vi "ALTS-2015 OPC Engine Main.vi"(8 "error in (no error)":errorcluster) -> (0 "error out":errorcluster)   [LabVIEW 2013]
doc: "Copyright © 2005, Soliton Technologies.\nAll rights reserved."
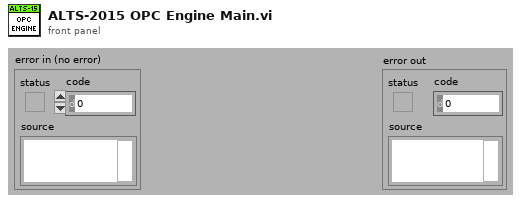
[diagram p1: front panel]
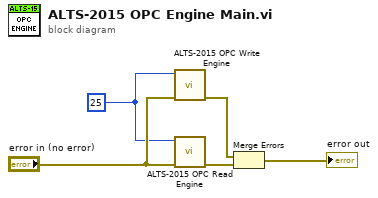
[diagram p0: block diagram]
diagram:
  w1 = u32 25 ("Delay (ms)")
  n1 = call "ALTS-2015 OPC Write Engine.vi"("error in (no error)"="error in (no error)", "Delay (ms)"=w1) -> ("error out"=w4:errorcluster)  [unwired: 9 in]
  n2 = call "ALTS-2015 OPC Read Engine.vi"("error in (no error)"="error in (no error)", "Delay (ms)"=w1) -> ("error out"=w5:errorcluster)  [unwired: 9 in]
  n3 = Merge Errors(w4, w5) -> (→"error out":errorcluster)
